vi "F Dwf Device Trigger Get.vi"(8 "error in (no error)":errorcluster, 9 "ptrigsrc":string, 10 "idxPin":i32, 11 "hdwf":i32) -> (0 "error out":errorcluster, 1 "ptrigsrc out":string, 3 "function return":i32)   [LabVIEW 2019, in "Olasdwf.lvlib"]
doc: "DWFAPI int FDwfDeviceTriggerGet(HDWF hdwf, int idxPin, TRIGSRC *ptrigsrc);"
uses:
  Olasdwf.lvlib
  Windows/System32/dwf.dll
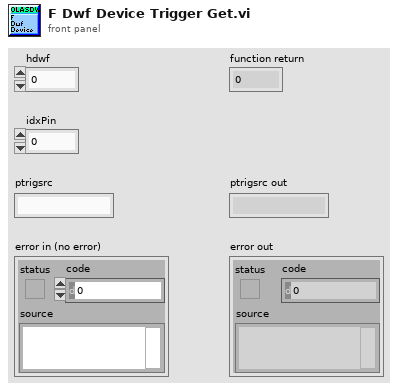
[diagram p1: front panel]
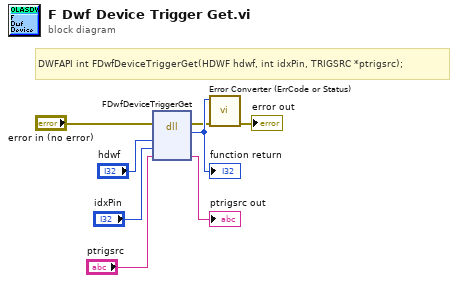
[diagram p0: block diagram]
diagram:
  # "DWFAPI int FDwfDeviceTriggerGet(HDWF hdwf, int idxPin, TRIGSRC *ptrigsrc);"
  n1 = dll-call lib="C:/Windows/System32/dwf.*" fn="FDwfDeviceTriggerGet"(error in="error in (no error)", "hdwf"="hdwf", "idxPin"="idxPin", "ptrigsrc"="ptrigsrc") -> (error out=w2:errorcluster, w8:i32, "ptrigsrc"=→"ptrigsrc out":string)  [unwired: 4 in, 1 out]
  "function return" <- w8
  n2 = call "Error Converter (ErrCode or Status).vi"("error in (no error)"=w2, "error code"=w8) -> ("error out"=→"error out":errorcluster)  [unwired: 9 in]
